vi "SeCrTs-Update PPSU Settings.vi"(8 "Error in":errorcluster, 11 "Cluster":T1) -> (0 "Fehler (Ausgang)":errorcluster caption="Error out")   [LabVIEW 2022 SP3]
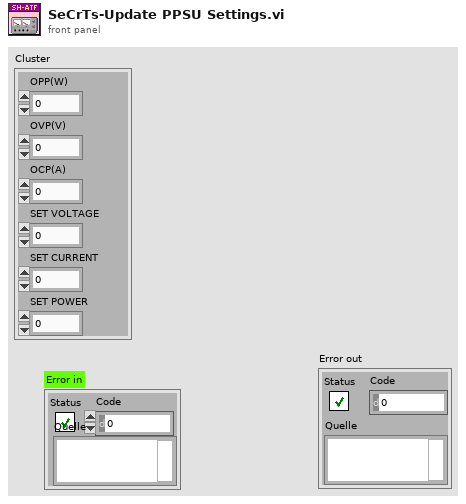
[diagram p1: front panel]
types:
  T1 = cluster{"OPP(W)":dbl, "OVP(V)":dbl, "OCP(A)":dbl, "SET VOLTAGE":dbl, "SET CURRENT":dbl, "SET POWER":dbl}
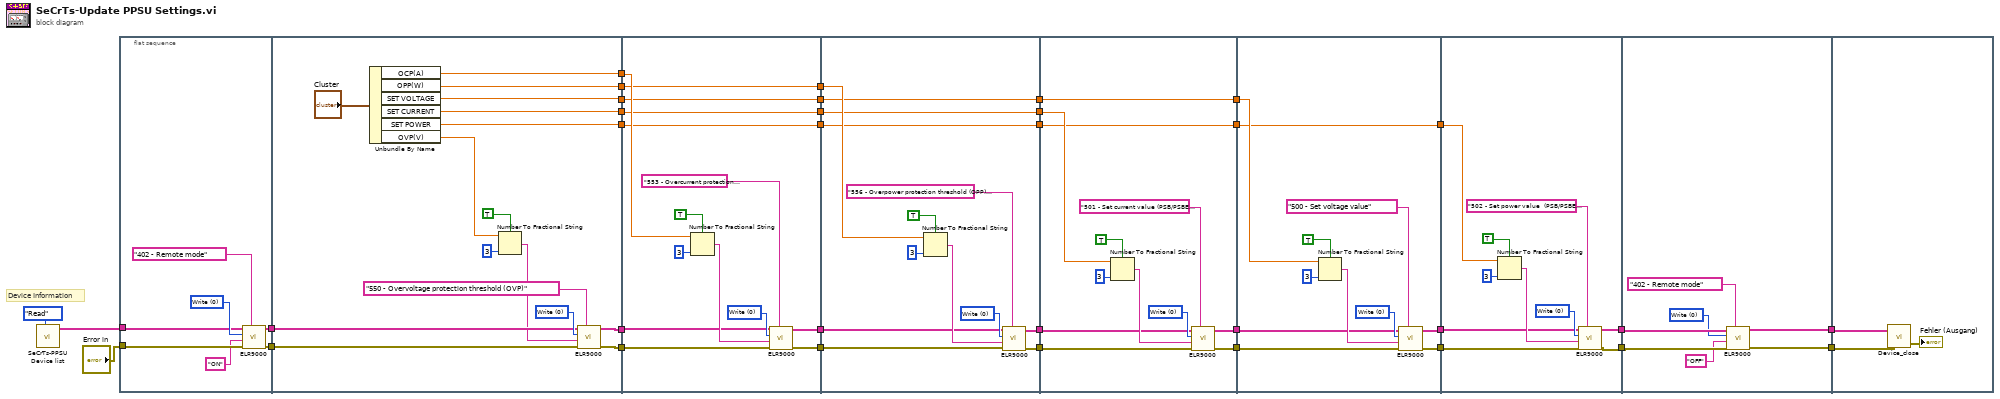
[diagram p0: block diagram]
diagram:
  # "Device Information"
  n1 = call "SeCrTs-PPSU Device list.vi"("Enum"=enum16{"Read", "Write"}."Read") -> ("Device information arrayR"=w1:string[])  [unwired: 9 in, 1 out]
  n2 = flat-sequence {
    tunnel: "Error in" -> [w41]
    tunnel: w1 -> [w35]
    tunnel: [w37] -> w34
    tunnel: [w36] -> w33
    tunnel: [w55] -> w32
    tunnel: [w54] -> w31
    tunnel: w34 -> [w53]
    tunnel: w33 -> [w52]
    tunnel: [w48] -> w30
    tunnel: [w47] -> w29
    tunnel: [w46] -> w28
    tunnel: [w45] -> w27
    tunnel: [w44] -> w26
    tunnel: w32 -> [w65]
    tunnel: w31 -> [w66]
    tunnel: [w64] -> w25
    tunnel: [w63] -> w24
    tunnel: w30 -> [w62]
    tunnel: [w61] -> w23
    tunnel: w29 -> [w61]
    tunnel: [w60] -> w22
    tunnel: w28 -> [w60]
    tunnel: [w59] -> w21
    tunnel: w27 -> [w59]
    tunnel: [w58] -> w20
    tunnel: w26 -> [w58]
    tunnel: w25 -> [w79]
    tunnel: w24 -> [w78]
    tunnel: [w77] -> w19
    tunnel: [w76] -> w18
    tunnel: w23 -> [w75]
    tunnel: [w74] -> w17
    tunnel: w22 -> [w74]
    tunnel: [w73] -> w16
    tunnel: w21 -> [w73]
    tunnel: [w72] -> w15
    tunnel: w20 -> [w72]
    tunnel: [w95] -> w14
    tunnel: [w94] -> w13
    tunnel: w19 -> [w89]
    tunnel: w18 -> [w88]
    tunnel: w17 -> [w87]
    tunnel: [w86] -> w12
    tunnel: w16 -> [w86]
    tunnel: [w85] -> w11
    tunnel: w15 -> [w85]
    tunnel: w14 -> [w100]
    tunnel: [w102] -> w10
    tunnel: w13 -> [w99]
    tunnel: [w101] -> w9
    tunnel: w12 -> [w98]
    tunnel: [w97] -> w8
    tunnel: w11 -> [w97]
    tunnel: w10 -> [w112]
    tunnel: [w110] -> w7
    tunnel: w9 -> [w111]
    tunnel: [w109] -> w6
    tunnel: w8 -> [w108]
    tunnel: w7 -> [w121]
    tunnel: [w122] -> w5
    tunnel: w6 -> [w124]
    tunnel: [w123] -> w4
    tunnel: w5 -> [w126]
    tunnel: w4 -> [w125]
    frame #0 {
      w39 = u8 0 items=["Write", "Read"] ("Access")
      n3 = call <instrlib>:"ELR9000.vi"("Command list"="402 - Remote mode", "Error in"=w41, "Value"="ON", "Access"=w39, "Device information in"=w35) -> ("Error out"=w36:errorcluster, "Device information out"=w37:string[])  [unwired: 1 in, 2 out]
    }
    frame #1 {
      w57 = u8 0 items=["Write", "Read"] ("Access")
      n4 = Unbundle By Name("Cluster") -> ("OCP(A)"=w48:dbl, "OPP(W)"=w47:dbl, "SET VOLTAGE"=w45:dbl, "SET CURRENT"=w46:dbl, "SET POWER"=w44:dbl, "OVP(V)"=w43:dbl)
      n5 = Number To Fractional String(use system decimal point (T)=TRUE, number=w43, precision (6)=i16 3) -> (F-format string=w49:string)  [unwired: 1 in]
      n6 = call <instrlib>:"ELR9000.vi"("Command list"="550 - Overvoltage protection threshold (OVP)", "Error in"=w52, "Value"=w49, "Access"=w57, "Device information in"=w53) -> ("Error out"=w55:errorcluster, "Device information out"=w54:string[])  [unwired: 1 in, 2 out]
    }
    frame #2 {
      w71 = u8 0 items=["Write", "Read"] ("Access")
      n7 = Number To Fractional String(use system decimal point (T)=TRUE, number=w62, precision (6)=i16 3) -> (F-format string=w67:string)  [unwired: 1 in]
      n8 = call <instrlib>:"ELR9000.vi"("Command list"="553 - Overcurrent protection threshold (OCP) (PSB/PSBE devices: source mode)", "Error in"=w65, "Value"=w67, "Access"=w71, "Device information in"=w66) -> ("Error out"=w63:errorcluster, "Device information out"=w64:string[])  [unwired: 1 in, 2 out]
    }
    frame #3 {
      w84 = u8 0 items=["Write", "Read"] ("Access")
      n9 = Number To Fractional String(use system decimal point (T)=TRUE, number=w75, precision (6)=i16 3) -> (F-format string=w80:string)  [unwired: 1 in]
      n10 = call <instrlib>:"ELR9000.vi"("Command list"="556 - Overpower protection threshold (OPP) (PSB/PSBE devices: source mode)", "Error in"=w78, "Value"=w80, "Access"=w84, "Device information in"=w79) -> ("Error out"=w76:errorcluster, "Device information out"=w77:string[])  [unwired: 1 in, 2 out]
    }
    frame #4 {
      w96 = u8 0 items=["Write", "Read"] ("Access")
      n11 = Number To Fractional String(use system decimal point (T)=TRUE, number=w87, precision (6)=i16 3) -> (F-format string=w90:string)  [unwired: 1 in]
      n12 = call <instrlib>:"ELR9000.vi"("Command list"="501 - Set current value (PSB/PSBE devices: source mode) / Irradiation (PV function, PSI/PSB only) ", "Error in"=w88, "Value"=w90, "Access"=w96, "Device information in"=w89) -> ("Error out"=w94:errorcluster, "Device information out"=w95:string[])  [unwired: 1 in, 2 out]
    }
    frame #5 {
      w107 = u8 0 items=["Write", "Read"] ("Access")
      n13 = Number To Fractional String(use system decimal point (T)=TRUE, number=w98, precision (6)=i16 3) -> (F-format string=w103:string)  [unwired: 1 in]
      n14 = call <instrlib>:"ELR9000.vi"("Command list"="500 - Set voltage value", "Error in"=w99, "Value"=w103, "Access"=w107, "Device information in"=w100) -> ("Error out"=w101:errorcluster, "Device information out"=w102:string[])  [unwired: 1 in, 2 out]
    }
    frame #6 {
      w117 = u8 0 items=["Write", "Read"] ("Access")
      n15 = Number To Fractional String(use system decimal point (T)=TRUE, number=w108, precision (6)=i16 3) -> (F-format string=w113:string)  [unwired: 1 in]
      n16 = call <instrlib>:"ELR9000.vi"("Command list"="502 - Set power value  (PSB/PSBE devices: source mode)", "Error in"=w111, "Value"=w113, "Access"=w117, "Device information in"=w112) -> ("Error out"=w109:errorcluster, "Device information out"=w110:string[])  [unwired: 1 in, 2 out]
    }
    frame #7 {
      w119 = u8 0 items=["Write", "Read"] ("Access")
      n17 = call <instrlib>:"ELR9000.vi"("Command list"="402 - Remote mode", "Error in"=w124, "Value"="OFF", "Access"=w119, "Device information in"=w121) -> ("Error out"=w123:errorcluster, "Device information out"=w122:string[])  [unwired: 1 in, 2 out]
    }
    frame #8 {
      n18 = call <instrlib>:"Device_close.vi"("error in (no error)"=w125, "Device information in"=w126) -> ("Fehler (Ausgang)"=→"Fehler (Ausgang)":errorcluster)  [unwired: 3 in]
    }
  }
